vi "GetDigitalPosition.vi"(0 "Handle":u32, 1 "Controller Channel":i32) -> (7 "FT_Status":u32(ring) items=["FT_OK", "FT_INVALID_HANDLE", "FT_DEVICE_NOT_FOUND", "FT_DEVICE_NOT_OPENED", "FT_IO_ERROR", "FT_INSUFFICIENT_RESOURCES", "FT_INVALID_PARAMETER", "FT_INVALID_BAUD_RATE", "FT_DEVICE_NOT_OPENED_FOR_ERASE", "FT_DEVICE_NOT_OPENED_FOR_WRITE", "FT_FAILED_TO_WRITE_DEVICE", "FT_EEPROM_READ_FAILED", "FT_EEPROM_WRITE_FAILED", "FT_EEPROM_ERASE_FAILED", "FT_EEPROM_NOT_PRESENT", "FT_EEPROM_NOT_PROGRAMMED", "FT_INVALID_ARGS", "FT_NOT_SUPPORTED", "FT_OTHER_ERROR"], 9 "Position":i32)   [LabVIEW 2013]
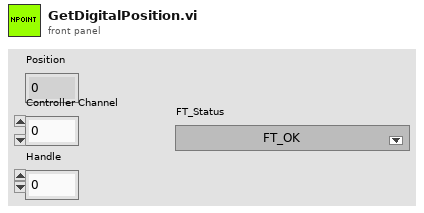
[diagram p1: front panel]
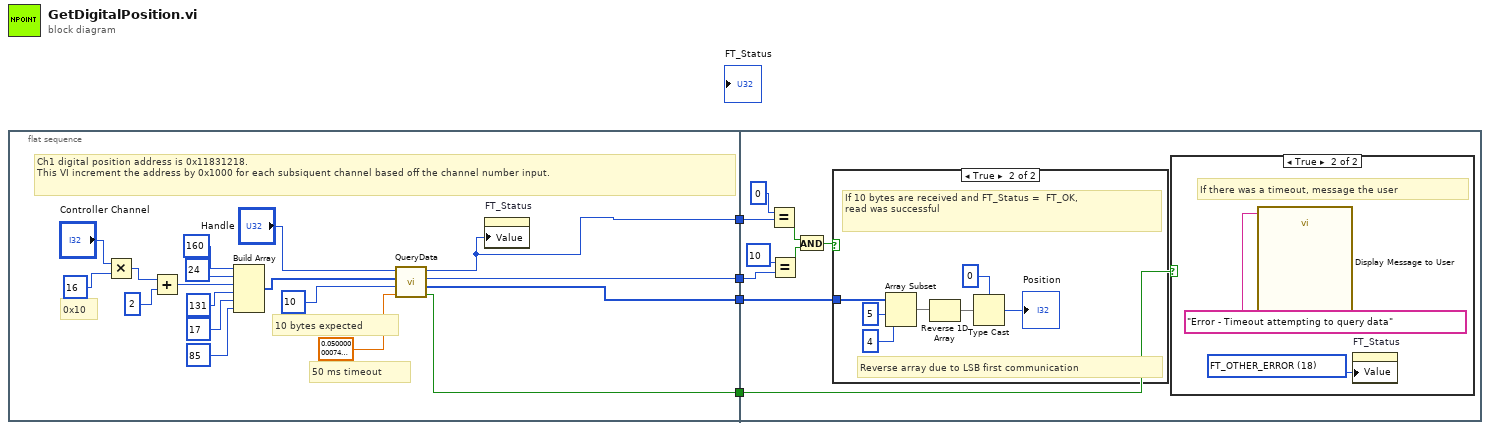
[diagram p0: block diagram]
diagram:
  n1 = flat-sequence {
    tunnel: [w8] -> w4
    tunnel: [w7] -> w3
    tunnel: [w6] -> w2
    tunnel: [w5] -> w1
    tunnel: w4 -> [w31]
    tunnel: w3 -> [w29]
    tunnel: w2 -> [w28]
    tunnel: w1 -> [w26]
    frame #0 {
      # "10 bytes expected"
      # "50 ms timeout"
      # "Ch1 digital position address is 0x11831218.\nThis VI increment the address by 0x1000 for each subsiquent channel based off the channel number input."
      # "0x10"
      n2 = Multiply(x="Controller Channel", y=u8 16) -> (x*y=w15:i32)
      n3 = Add(x=w15, y=u8 2 ("element")) -> (x+y=w14:i32)
      n4 = Build Array(u8 160 ("element"), u8 24 ("element"), w14, u8 131 ("element"), u8 17 ("element"), u8 85 ("element")) -> (w11:i32[])
      n5 = call "QueryData.vi"("TimeoutLengthSeconds"=sgl 0.05, "NumBytesExpected"=u32 10, "Message"=w11, "Handle"="Handle") -> ("Timeout"=w6:bool, "Return Array"=w7:u8[], "Bytes Read"=w8:u32, "FT_Status"=w5:u32)  [unwired: 4 in]
      n6 = property on="FT_Status" class="Ring (strict)"("Value"=w5) -> ()  [unwired: 2 in, 2 out]
    }
    frame #1 {
      n7 = Equal?(x=u32 0, y=w26) -> (x = y?=w24:bool)
      n8 = Equal?(x=u32 10, y=w31) -> (x = y?=w25:bool)
      n9 = And(x=w24, y=w25) -> (x .and. y?=w23:bool)
      n10 = case shown="True" w23 {
        tunnel: w29 -> [_ w40]
        frame False {
        }
        frame True {
          # "Reverse array due to LSB first communication"
          # "If 10 bytes are received and FT_Status =  FT_OK,\nread was successful"
          n11 = Array Subset(array=w40, index=5, length=4) -> (w36:u8[])
          n12 = Reverse 1D Array(array=w36) -> (reversed array=w35:u8[])
          n13 = Type Cast(type=0, x=w35) -> (*(type *) &x=→"Position":i32)
        }
      }
      n14 = case shown="True" w28 {
        frame False {
        }
        frame True {
          w32 = u32 18 items=["FT_OK", "FT_INVALID_HANDLE", "FT_DEVICE_NOT_FOUND", "FT_DEVICE_NOT_OPENED", "FT_IO_ERROR", "FT_INSUFFICIENT_RESOURCES", "FT_INVALID_PARAMETER", "FT_INVALID_BAUD_RATE", "FT_DEVICE_NOT_OPENED_FOR_ERASE", "FT_DEVICE_NOT_OPENED_FOR_WRITE", "FT_FAILED_TO_WRITE_DEVICE", "FT_EEPROM_READ_FAILED", "FT_EEPROM_WRITE_FAILED", "FT_EEPROM_ERASE_FAILED", "FT_EEPROM_NOT_PRESENT", "FT_EEPROM_NOT_PROGRAMMED", "FT_INVALID_ARGS", "FT_NOT_SUPPORTED", "FT_OTHER_ERROR"] ("FT_Status")
          # "If there was a timeout, message the user"
          n15 = call "Display Message to User"("Message"="Error - Timeout attempting to query data") -> ()  [unwired: 9 in, 2 out]
          n16 = property on="FT_Status" class="Ring (strict)"("Value"=w32) -> ()  [unwired: 2 in, 2 out]
        }
      }
    }
  }
